vi "Trim Whitespace__JDP.vi"(5 "Remove (leading and trailing)":enum16{"leading", "trailing", "both"}(ring)=enum."both", 6 "String in":string) -> (1 "String out":string)   [LabVIEW 2019, in "JDP Utility.lvlib"]
doc: "Removes leading and/or trailing whitespace from a string.\nWhitespace is defined as any of the following characters (where values are in the format: dec, hex, string):\n <b>tab</b> = 9, 0x09, \\t\n <b>newline</b> = 10, 0x0A, \\n\n <b>vertical tab</b> = 11, 0x0B, \\0B\n <b>form feed</b> = 12, 0x0C, \\f\n <b>carriage return</b> = 13, 0x0D, \\r \n <b>space</b> = 32, 0x20, \\s"
uses:
  JDP Utility.lvlib
panel:
  # "VI copied from OpenG:\n-- converted to inlined from subroutine preallocate reentrant\n-- force serialization of leading and trailing"
  # "Trim Whitespace (String) 1.vi\n\nRemoves leading and/or trailing whitespace from a string.\n\nPlease visit http://www.OpenG.org to learn about the\nOpen Source LabVIEW software movement.\n\nNOTICE -- YOU MUST LEAVE THIS NOTICE IN PLACE.  PER THE TERMS OF THE LICENSE BELOW, YOU MAY SUBLICENSE THIS SOFTWARE \nIN ANY WAY THAT DOES NOT CONFLICT WITH THIS LICENSE.\n\n### BSD License (http://www.opensource.org/licenses/bsd-license.php) Begin ###\n\nCopyright (c) 2002-2006, Jim Kring <jim@jimkring.com>\nCopyright (c) 2002, Cal-Bay Systems, Inc. <info@calbay.com>\nCopyright (c) 2011,  Shaun Rumbell <shaunr@labview-tools.com> \nCopyright (c) 2011,  Darin.K <darin@alum.mit.edu>\nCopyright (c) 2011, Jonathon Green <jg@jgcode.net>\n\nAll rights reserved.\n\nRedistribution and use in source and binary forms, with or without modification, are permitted provided that the following conditions are met:\n\n    * Redistributions of source code must retain the above copyright notice, this list of conditions and the following disclaimer.\n    * Redistributions in binary form must reproduce the above copyright notice, this list of conditions and the following disclaimer in the \n       documentation and/or other materials provided with the distribution.\n    * Neither the name of SciWare, James Kring, Inc., nor the names of its contributors may be used to endorse or promote products derived \n       from this software without specific prior written permission.\n\nTHIS SOFTWARE IS PROVIDED BY THE COPYRIGHT HOLDERS AND CONTRIBUTORS \"AS IS\" AND ANY EXPRESS OR IMPLIED WARRANTIES, \nINCLUDING, BUT NOT LIMITED TO, THE IMPLIED WARRANTIES OF MERCHANTABILITY AND FITNESS FOR A PARTICULAR PURPOSE ARE \nDISCLAIMED. IN NO EVENT SHALL THE COPYRIGHT OWNER OR CONTRIBUTORS BE LIABLE FOR ANY DIRECT, INDIRECT, INCIDENTAL,\n SPECIAL, EXEMPLARY, OR CONSEQUENTIAL DAMAGES (INCLUDING, BUT NOT LIMITED TO, PROCUREMENT OF SUBSTITUTE GOODS OR \nSERVICES; LOSS OF USE, DATA, OR PROFITS; OR BUSINESS INTERRUPTION) HOWEVER CAUSED AND ON ANY THEORY OF LIABILITY, \nWHETHER IN CONTRACT, STRICT LIABILITY, OR TORT (INCLUDING NEGLIGENCE OR OTHERWISE) ARISING IN ANY WAY OUT OF THE USE \nOF THIS SOFTWARE, EVEN IF ADVISED OF THE POSSIBILITY OF SUCH DAMAGE.\n\n### BSD License End ###"
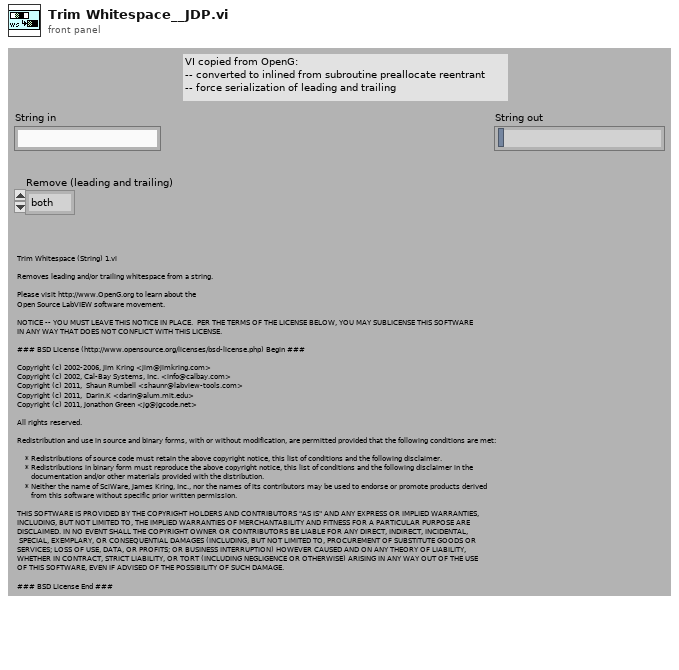
[diagram p1: front panel]
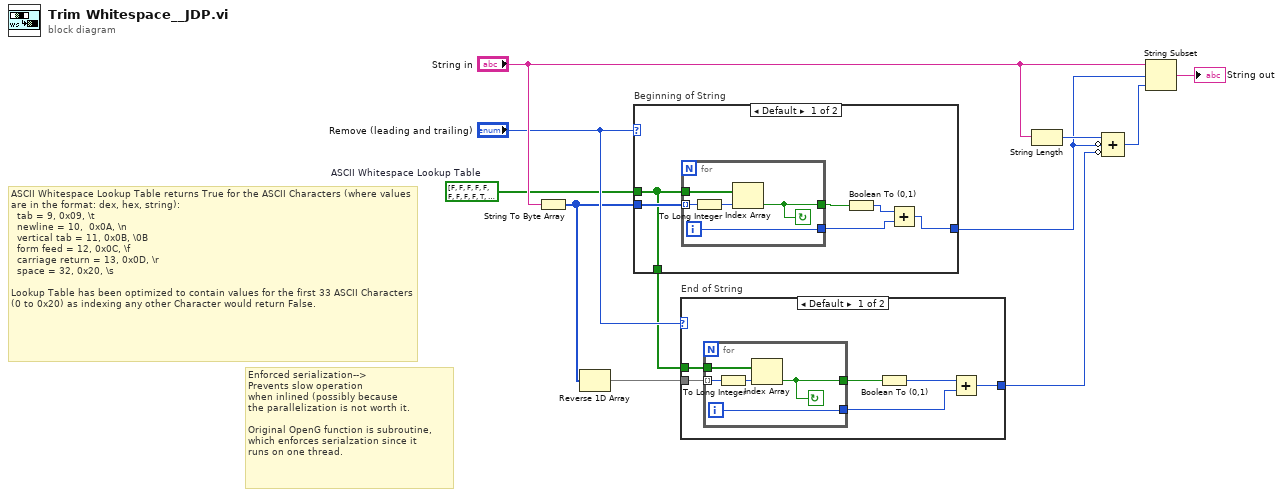
[diagram p0: block diagram]
diagram:
  w2 = bool[] [FALSE, FALSE, FALSE, FALSE, FALSE, FALSE, FALSE, FALSE, FALSE, TRUE, TRUE, TRUE, TRUE, TRUE, FALSE, FALSE, FALSE, FALSE, FALSE, FALSE, FALSE, FALSE, FALSE, FALSE, FALSE, FALSE, FALSE, FALSE, FALSE, FALSE, FALSE, FALSE, TRUE]  # ASCII Whitespace Lookup Table
  # "Enforced serialization-->\nPrevents slow operation \nwhen inlined (possibly because\nthe parallelization is not worth it.\n\nOriginal OpenG function is subroutine,\nwhich enforces serialzation since it\nruns on one thread."
  # "ASCII Whitespace Lookup Table returns True for the ASCII Characters (where values are in the format: dex, hex, string):\n  tab = 9, 0x09, \\t\n  newline = 10,  0x0A, \\n\n  vertical tab = 11, 0x0B, \\0B\n  form feed = 12, 0x0C, \\f\n  carriage return = 13, 0x0D, \\r \n  space = 32, 0x20, \\s\n\nLookup Table has been optimized to contain values for the first 33 ASCII Characters (0 to 0x20) as indexing any other Character would return False."
  n1 = String To Byte Array(string="String in") -> (unsigned byte array=w4:u8[])
  n2 = Reverse 1D Array(array=w4) -> (reversed array=w10:u8[])
  n3 = case "Beginning of String" shown="Default" "Remove (leading and trailing)" {
    tunnel: w4 -> [w17 _]
    tunnel: [w12 _] -> w3
    tunnel: w2 -> [w16 w23]
    tunnel: [w16 w23] -> w1
    frame Default {
      n4 = for {
        tunnel: w17 -> [w20] mode=indexing
        tunnel: [w22] -> w13
        tunnel: w16 -> [w21]
        tunnel: [w18] -> w14
        i -> [w22]
        stop <- w18 continue-if-true
        n5 = To Long Integer(number=w20) -> (32bit integer=w19:i32)
        n6 = Index Array(array=w21, index=w19) -> (element=w18:bool)
      }
      n7 = Boolean To (0,1)(Boolean=w14) -> (0, 1=w15:i16)
      n8 = Add(x=w15, y=w13) -> (x+y=w12:i32)
    }
    frame "trailing" {
    }
  }
  n9 = case "End of String" shown="Default" "Remove (leading and trailing)" {
    tunnel: w10 -> [w29 _]
    tunnel: [w27 _] -> w5
    tunnel: w1 -> [w26 _]
    frame Default {
      n10 = for {
        tunnel: w29 -> [w31] mode=indexing
        tunnel: [w34] -> w28
        tunnel: [w32] -> w25
        tunnel: w26 -> [w33]
        i -> [w34]
        stop <- w32 continue-if-true
        n11 = To Long Integer(number=w31) -> (32bit integer=w30:i32)
        n12 = Index Array(array=w33, index=w30) -> (element=w32:bool)
      }
      n13 = Boolean To (0,1)(Boolean=w25) -> (0, 1=w24:i16)
      n14 = Add(x=w24, y=w28) -> (x+y=w27:i32)
    }
    frame "leading" {
    }
  }
  n15 = String Length(string="String in") -> (length=w8:i32)
  n16 = Compound Arithmetic op=ADD(w8, invert w3, invert w5) -> (w9:i32)
  n17 = String Subset(string="String in", offset (0)=w3, length (rest)=w9) -> (substring=→"String out":string)
